vi "InitializeFlagData.vi"(8 "inputError":errorcluster, 10 "inputPath":string) -> (0 "outputError":errorcluster, 2 "outputFlagData":T1)   [LabVIEW 2020]
uses:
  CommonControl/Flag.ctl
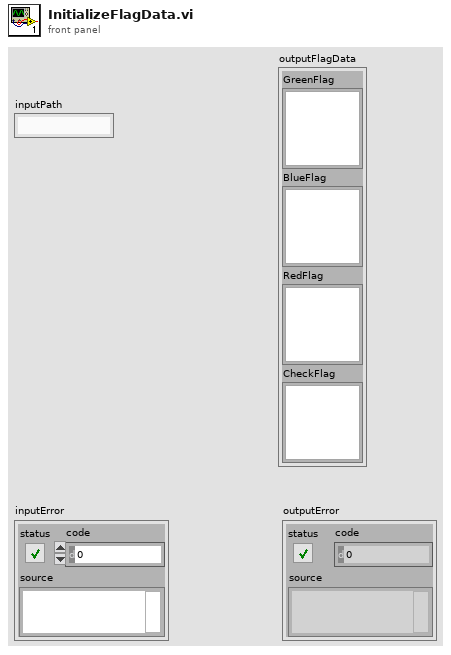
[diagram p1: front panel]
types:
  T1 = typedef "Flag.ctl" = cluster{"GreenFlag":picture, "BlueFlag":picture, "RedFlag":picture, "CheckFlag":picture}
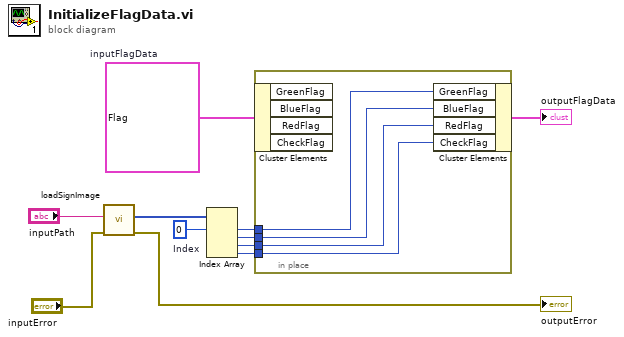
[diagram p0: block diagram]
diagram:
  w11 = T1 {"GreenFlag"=bytes[0], "BlueFlag"=bytes[0], "RedFlag"=bytes[0], "CheckFlag"=bytes[0]}  # inputFlagData
  w7 = 0  # Index
  n1 = call "loadSignImage.vi"("inputError"="inputError", "String"="inputPath") -> ("outputError"=→"outputError":errorcluster, "SignImageOutput"=w1:picture[])  [unwired: 8 in]
  n2 = Index Array "Index Array"(array=w1, index #1=w7) -> (element #1=w8:picture, element #2=w9:picture, element #3=w10:picture, element #4=w3:picture)  [unwired: 3 in]
  n3 = in-place {
    in-place-border: w8 -> [w15]
    in-place-border: w9 -> [w14]
    in-place-border: w10 -> [w13]
    in-place-border: w3 -> [w12]
    n4 = in-place-cluster #1(w11) -> ()  [unwired: 4 out]
    n5 = in-place-cluster #1("GreenFlag"=w15, "BlueFlag"=w14, "RedFlag"=w13, "CheckFlag"=w12) -> (→"outputFlagData":T1)
  }
